vi "lab3.vi"() -> ()   [LabVIEW 2010]
panel:
  in  "Количество\nэлементов\nподмножества":i32
  in  "Старт\nподмножества":i32
  in  "Масштабный\nкоэффициент":dbl
  out "Конечный массив":dbl[](array[numeric])
  out "Подмножество массива":dbl[](array[numeric])
  out "Массив случайных чисел":dbl[](array[numeric])
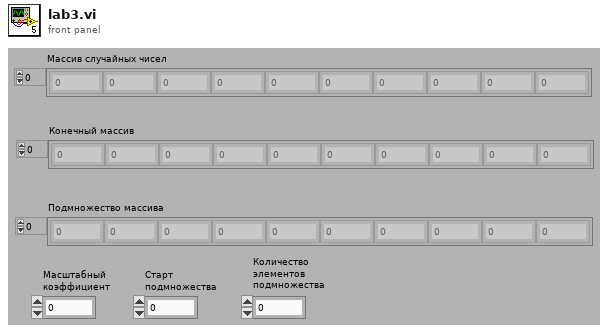
[diagram p1: front panel]
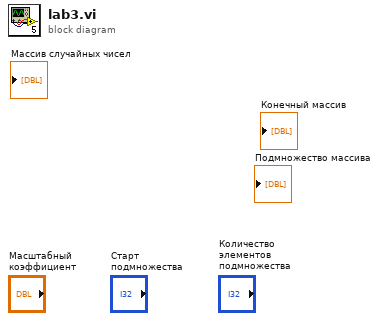
[diagram p0: block diagram]
diagram:
